vi "Register gRPC Methods.vi"(8 "error in (no error)":errorcluster, 11 "gRPC service in":refnum<class "OOBgRPCService.lvclass">) -> (0 "error out":errorcluster, 3 "gRPC service out":refnum<class "OOBgRPCService.lvclass">)   [LabVIEW 2025, in "OOB gRPC Server.lvlib" / "OOBgRPCService.lvclass"]
uses:
  OOBgRPCService.lvclass
  typeDefs/Server Internal UEs.ctl
  typeDefs/Server Internal Message.ctl
  typeDefs/Server gRPC UEs.ctl
  <vilib>/gRPC/LabVIEW gRPC Library/Server API/typeDefs/gRPCId Cluster.ctl
  <vilib>/gRPC/LabVIEW gRPC Library/Shared/grpcId.ctl
  OOBgRPCService.lvclass/OOBgRPCService.ctl
  <vilib>/gRPC/LabVIEW gRPC Library/grpc-lvsupport-release.lvlib
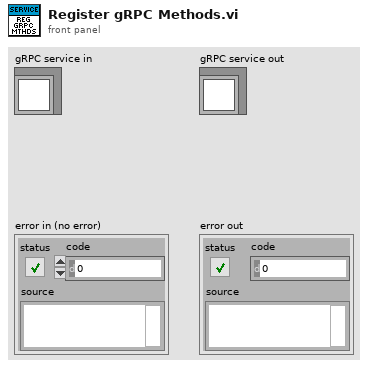
[diagram p1: front panel]
types:
  T1 = typedef "OOB gRPC Server.lvlib/OOBgRPCService.lvclass/Server gRPC UEs.ctl" = cluster{"OOBgRPCService Generic gRPC UE":refnum<user-event>, "OOBgRPCService PauseResume gRPC UE":refnum<user-event>, "OOBgRPCService Export gRPC UE":refnum<user-event>}
  T2 = typedef "OOB gRPC Server.lvlib/OOBgRPCService.lvclass/Server Internal UEs.ctl" = cluster{"OOBgRPCService Generic Internal UE":refnum<user-event>, "OOBgRPCService PauseResume Internal UE":refnum<user-event>, "OOBgRPCService Export Internal UE":refnum<user-event>}
  T3 = typedef "grpc-lvsupport-release.lvlib/grpcId.ctl" = u64
  T4 = typedef "OOB gRPC Server.lvlib/OOBgRPCService.lvclass/Server Internal Message UE.ctl" = refnum<user-event>
  T5 = typedef "grpc-lvsupport-release.lvlib/gRPCId Cluster UE.ctl" = refnum<user-event>
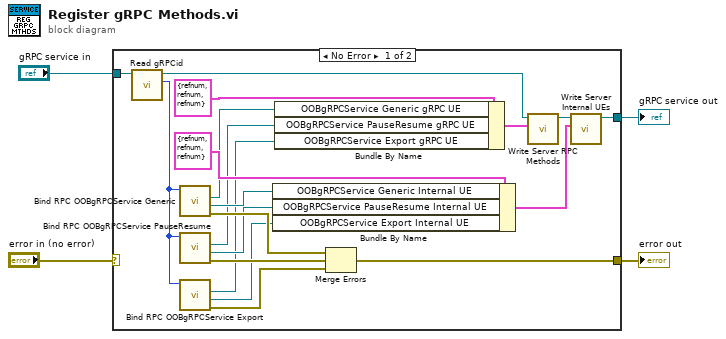
[diagram p0: block diagram]
diagram:
  n1 = case shown="No Error" "error in (no error)" {
    selector: "error in (no error)" -> [_ w24]
    tunnel: "gRPC service in" -> [w15 w25]
    tunnel: [w23 w24] -> w3
    tunnel: [w22 w25] -> w2
    frame No Error {
      n2 = call-dynamic "Read gRPCid.vi"("gRPC service in"=w15) -> ("gRPCid"=w14:T3, "gRPC service out"=w16:refnum<class "OOBgRPCService.lvclass">)  [unwired: 8 in, 1 out]
      n3 = call "Bind RPC OOBgRPCService Generic.vi"("gRPCid server in"=w14) -> ("error out"=w13:errorcluster, "OOBgRPCService Generic Internal UE"=w11:T4, "OOBgRPCService Generic gRPC UE"=w12:T5)  [unwired: 7 in, 1 out]
      n4 = call "Bind RPC OOBgRPCService PauseResume.vi"("gRPCid server in"=w14) -> ("error out"=w10:errorcluster, "OOBgRPCService PauseResume Internal UE"=w8:T4, "OOBgRPCService PauseResume gRPC UE"=w9:T5)  [unwired: 7 in, 1 out]
      n5 = call "Bind RPC OOBgRPCService Export.vi"("gRPCid server in"=w14) -> ("error out"=w7:errorcluster, "OOBgRPCService Export Internal UE"=w5:T4, "OOBgRPCService Export gRPC UE"=w6:T5)  [unwired: 7 in, 1 out]
      n6 = Bundle By Name ("Bundle Internal UEs")(cluster=T2 {"OOBgRPCService Generic Internal UE"=refnum, "OOBgRPCService PauseResume Internal UE"=refnum, "OOBgRPCService Export Internal UE"=refnum} ("Server Internal UEs"), "OOBgRPCService Generic Internal UE"=w11, "OOBgRPCService PauseResume Internal UE"=w8, "OOBgRPCService Export Internal UE"=w5) -> (w21:T2)
      n7 = Bundle By Name ("Bundle gRPC UEs")(cluster=T1 {"OOBgRPCService Generic gRPC UE"=refnum, "OOBgRPCService PauseResume gRPC UE"=refnum, "OOBgRPCService Export gRPC UE"=refnum} ("gRPC Server Method Events"), "OOBgRPCService Generic gRPC UE"=w12, "OOBgRPCService PauseResume gRPC UE"=w9, "OOBgRPCService Export gRPC UE"=w6) -> (w18:T1)
      n8 = Merge Errors(w13, w10, w7) -> (w23:errorcluster)
      n9 = call "Write Server RPC Methods.vi"("Server RPC Methods"=w18, "gRPC service in"=w16) -> ("gRPC service out"=w19:refnum<class "OOBgRPCService.lvclass">)  [unwired: 8 in, 1 out]
      n10 = call "Write Server Internal UEs.vi"("Server Internal UEs"=w21, "gRPC service in"=w19) -> ("gRPC service out"=w22:refnum<class "OOBgRPCService.lvclass">)  [unwired: 8 in, 1 out]
    }
    frame Error {
    }
  }
  "error out" <- w3
  "gRPC service out" <- w2
